vi "Log ERROR.vi"(8 "error in (no error)":errorcluster, 11 "Message":string) -> (0 "error out":errorcluster)   [LabVIEW 2016, in "BTL_logger.lvlib"]
uses:
  BTL_logger.lvlib
  Levels.ctl
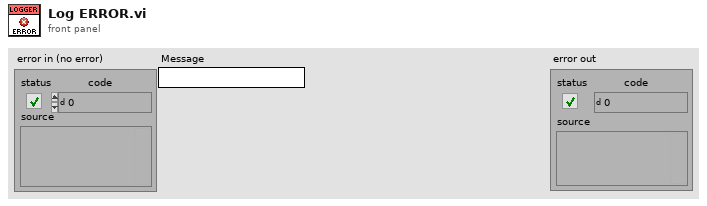
[diagram p1: front panel]
types:
  T1 = typedef "BTL_logger.lvlib/Levels.ctl" = enum16{"ALL", "TRACE", "DEBUG", "INFO", "WARN", "ERROR", "FATAL", "OFF"}
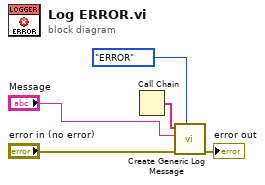
[diagram p0: block diagram]
diagram:
  n1 = Call Chain() -> (call chain=w1:string[])
  n2 = call "Create Generic Log Message.vi"("Level"=Levels."ERROR", "error in (no error)"="error in (no error)", "Message"="Message", "Call Chain"=w1) -> ("error out"=→"error out":errorcluster)  [unwired: 7 in]
